vi "rvc Map Example.vi"(11 "Array in":dbl[][](array[numeric])) -> (3 "Array out":dbl[][](array[numeric]))   [LabVIEW 2014]
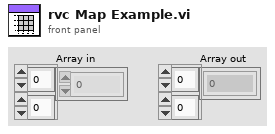
[diagram p1: front panel]
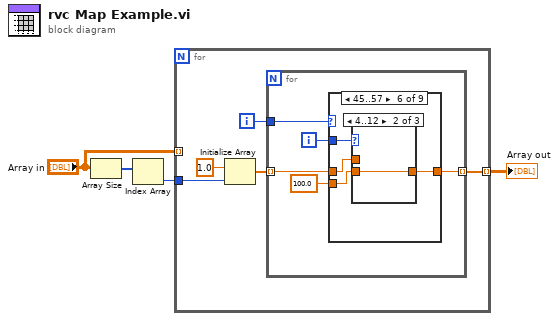
[diagram p0: block diagram]
diagram:
  n1 = Array Size(array="Array in") -> (size(s)=w2:i32[])
  n2 = Index Array(array=w2) -> (element=w1:i32)  [unwired: 1 in]
  n3 = for {
    tunnel: "Array in" -> [_] mode=indexing
    tunnel: [w9] -> w4 mode=indexing
    tunnel: w1 -> [w5]
    i -> [w6]
    n4 = Initialize Array(1.0 ("element"), w5) -> (w7:dbl[])
    n5 = for {
      tunnel: w7 -> [w14] mode=indexing
      tunnel: [w13] -> w9 mode=indexing
      tunnel: w6 -> [w10]
      i -> [w11]
      n6 = case shown="45..57" w10 {
        tunnel: [w15 w16 w18 w25 w31 w38 w45 w52 w58] -> w13
        tunnel: w14 -> [w15 w16 w17 w24 w33 w40 w47 w54 w59]
        tunnel: 100.0 ("element") -> [_ _ w19 w26 w32 w39 w46 w53 w60]
        tunnel: w11 -> [_ _ w20 w27 w30 w37 w44 w51 w61]
        frame 0, Default {
        }
        frame 1..6 {
        }
        frame 7..14 {
          n7 = case shown="59..66" w20 {
            tunnel: [w21 w22 w23] -> w18
            tunnel: w19 -> [_ w22 w23]
            tunnel: w17 -> [w21 _ _]
            frame 0, Default {
            }
            frame 4..12 {
            }
            frame 59..66 {
            }
          }
        }
        frame 15..22 {
          n8 = case shown="4..81" w27 {
            tunnel: [w28 w29] -> w25
            tunnel: w26 -> [_ w29]
            tunnel: w24 -> [w28 _]
            frame 0, Default {
            }
            frame 4..81 {
            }
          }
        }
        frame 23..44 {
          n9 = case shown="59..66" w30 {
            tunnel: [w34 w35 w36] -> w31
            tunnel: w32 -> [_ w35 w36]
            tunnel: w33 -> [w34 _ _]
            frame 0, Default {
            }
            frame 4..12 {
            }
            frame 59..66 {
            }
          }
        }
        frame 45..57 {
          n10 = case shown="4..12" w37 {
            tunnel: [w41 w42 w43] -> w38
            tunnel: w39 -> [_ w42 w43]
            tunnel: w40 -> [w41 _ _]
            frame 0, Default {
            }
            frame 4..12 {
            }
            frame 22..78 {
            }
          }
        }
        frame 58..68 {
          n11 = case shown="0, Default" w44 {
            tunnel: [w48 w49 w50] -> w45
            tunnel: w46 -> [_ w49 w50]
            tunnel: w47 -> [w48 _ _]
            frame 0, Default {
            }
            frame 4..12 {
            }
            frame 59..66 {
            }
          }
        }
        frame 69..78 {
          n12 = case shown="59..66" w51 {
            tunnel: [w55 w56 w57] -> w52
            tunnel: w53 -> [_ w56 w57]
            tunnel: w54 -> [w55 _ _]
            frame 0, Default {
            }
            frame 4..38 {
            }
            frame 59..66 {
            }
          }
        }
        frame 79..92 {
          n13 = case shown="59..66" w61 {
            tunnel: [w62 w63 w64] -> w58
            tunnel: w60 -> [_ w63 w64]
            tunnel: w59 -> [w62 _ _]
            frame 0, Default {
            }
            frame 4..12 {
            }
            frame 59..66 {
            }
          }
        }
      }
    }
  }
  "Array out" <- w4
